vi "RandomPointEnemyField.vi"(9 "Field defense":dbl[](array[numeric]), 10 "IA State Input":T1) -> (2 "Point Enemy Field":dbl[](array[numeric]))   [LabVIEW 2017]
uses:
  Core/AI Input.ctl
  Core/AI Robot.ctl
  Intel/Functions Enum.ctl
  Intel/AttackerStates.ctl
  Path Planning/RRT/PathDests.ctl
  Path Planning/RRT/PathDest.ctl
  Core/AI Ball.ctl
  Core/Field Size.ctl
  Core/AI Judge.ctl
  Intel/Command Enum.ctl
  Util/Events/Events.ctl
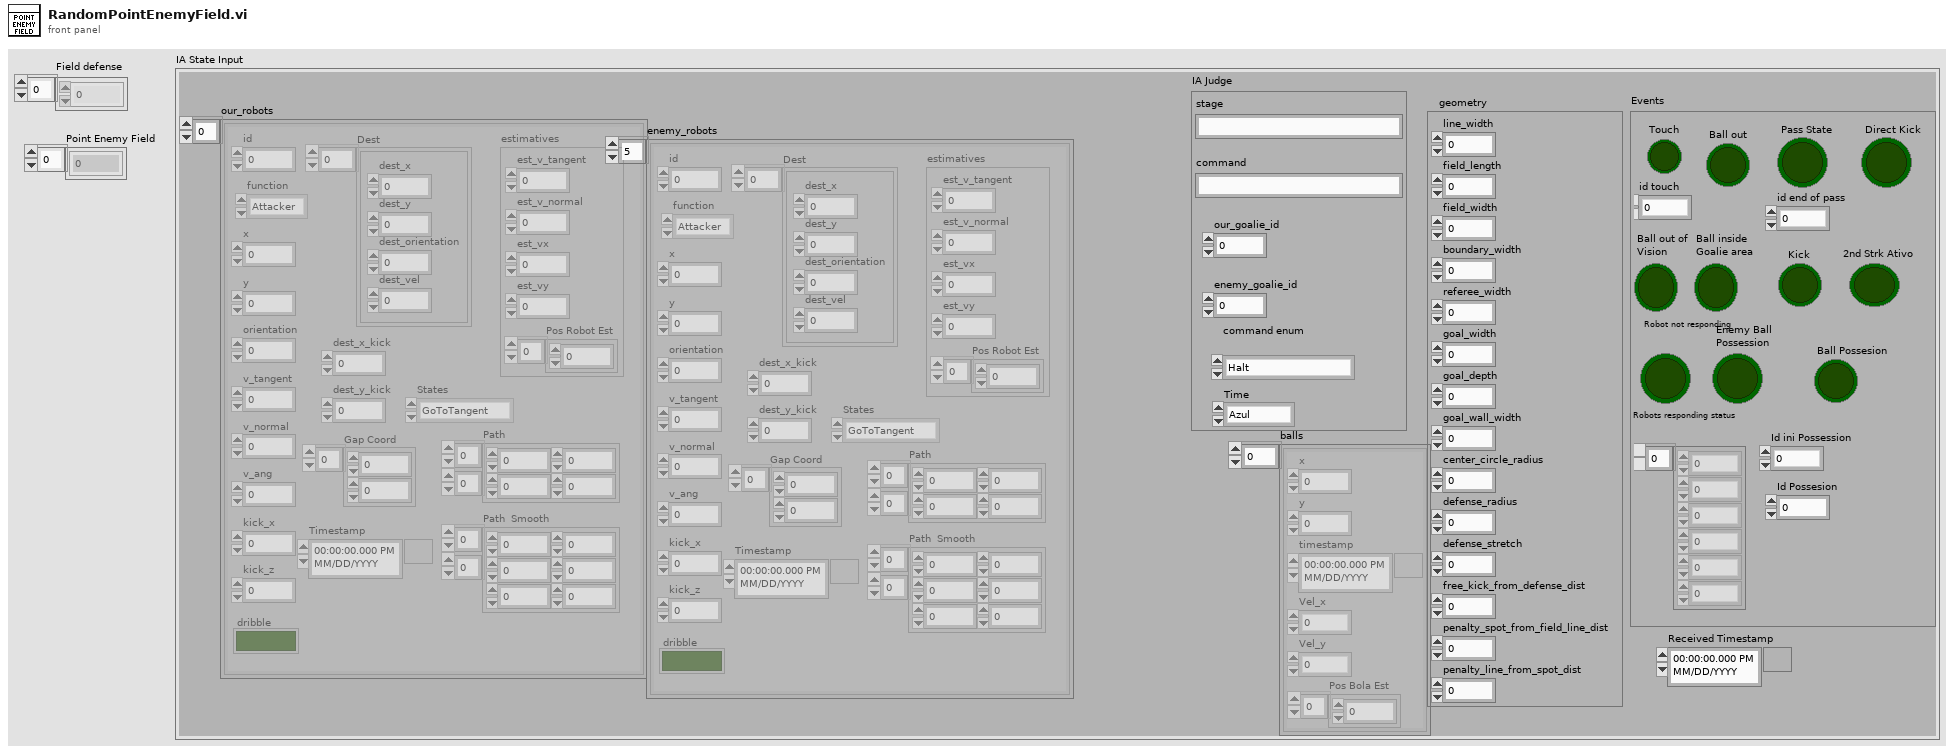
[diagram p1: front panel]
types:
  T1 = typedef "AI Input.ctl" = cluster{"our_robots":T2[], "enemy_robots":T2[], "balls":T7[], "geometry":T8, "IA Judge":T9, "Received Timestamp":timestamp, "Events":T11}
  T2 = typedef "AI Robot.ctl" = cluster{"id":u32, "function":T3, "x":dbl, "y":dbl, "orientation":dbl, "v_tangent":dbl, "v_normal":dbl, "v_ang":dbl, "kick_x":dbl, "kick_z":dbl, "dribble":bool, "Timestamp":timestamp, "estimatives":cluster{"est_v_tangent":dbl, "est_v_normal":dbl, "est_vx":dbl, "est_vy":dbl, "Pos Robot Est":dbl[]}, "dest_x_kick":dbl, "dest_y_kick":dbl, "Gap Coord":dbl[], "States":T4, "Path ":dbl[][], "Path  Smooth":dbl[][], "Dest":T5}
  T3 = typedef "Functions Enum.ctl" = enum16{"2nd Striker", "Attacker", "Goalie", "Defender", "Striker", "Goto 0", "Dummy", "Kicker", "ZigZag 0", "ZigZag 1", "ZigZag 2", "ZigZag 3", "ZigZag 4", "ZigZag 5", "ZigZag 6", "ZigZag 7", "ZigZag 8", ""}
  T4 = typedef "AttackerStates.ctl" = enum16{"Pass", "GoToTangent", "BallGetting", "GoToKick", ""}
  T5 = typedef "PathDests.ctl" = T6[]
  T6 = typedef "PathDest.ctl" = cluster{"dest_x":dbl, "dest_y":dbl, "dest_orientation":dbl, "dest_vel":dbl}
  T7 = typedef "AI Ball.ctl" = cluster{"x":dbl, "y":dbl, "timestamp":timestamp, "Vel_x":dbl, "Vel_y":dbl, "Pos Bola Est":dbl[]}
  T8 = typedef "Field Size.ctl" = cluster{"line_width":u32, "field_length":u32, "field_width":u32, "boundary_width":u32, "referee_width":u32, "goal_width":u32, "goal_depth":u32, "goal_wall_width":u32, "center_circle_radius":u32, "defense_radius":u32, "defense_stretch":u32, "free_kick_from_defense_dist":u32, "penalty_spot_from_field_line_dist":u32, "penalty_line_from_spot_dist":u32}
  T9 = typedef "AI Judge.ctl" = cluster{"stage":string, "command":string, "our_goalie_id":dbl, "enemy_goalie_id":dbl, "command enum":T10, "Time":enum16{"Azul", "Amarelo"}}
  T10 = typedef "Command Enum.ctl" = enum16{"Halt", "Stop", "Force Start", "PKA Normal Start", "Prepare Kickoff Ally", "PKE Normal Start", "Prepare Kickoff Enemy", "Prepare Penalty Ally", "PPA Normal Start", "Prepare Penalty Enemy", "PPE Normal Start", "Direct Free Enemy", "Direct Free Ally", "Indirect Free Enemy", "Indirect Free Ally", "Timeout Enemy", "Timeout Ally", "Goal Enemy", "Goal Ally", "Ball Placement Enemy", "Ball Placement Ally", "Normal Half Time", "Extra Time Break", "Extra Half Time", "None", "Post Game"}
  T11 = typedef "Events.ctl" = cluster{"Touch":bool, "Ball out":bool, "id touch":dbl, "Ball out of \nVision":bool, "Ball inside \nGoalie area":bool, "Robot not responding":bool, "Robots responding status":dbl[], "Enemy Ball \nPossession":bool, "Pass State":bool, "id end of pass":dbl, "Kick":bool, "Id ini Possession":dbl, "Ball Possesion":bool, "Id Possesion":dbl, "Direct Kick":bool, "2nd Strk Ativo":bool}
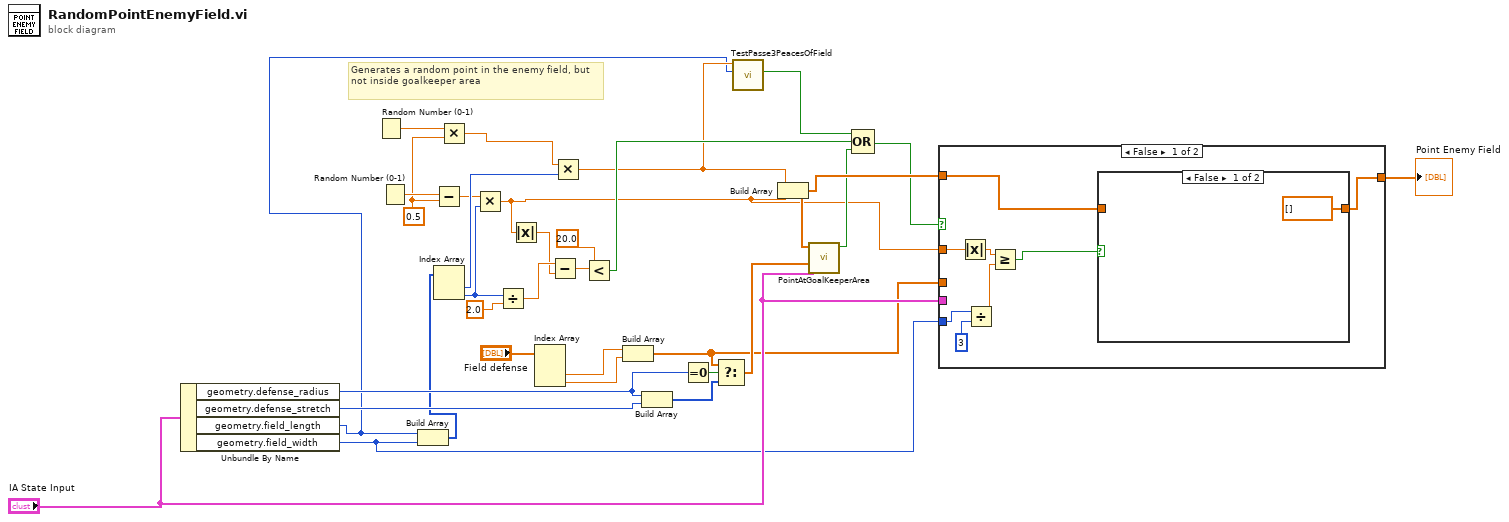
[diagram p0: block diagram]
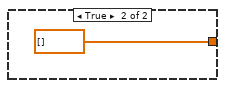
[diagram p3: hidden frame]
diagram:
  w29 = 0.5 ("y")
  # "Generates a random point in the enemy field, but not inside goalkeeper area"
  n1 = Unbundle By Name("IA State Input") -> ("geometry.defense_radius"=w14:u32, "geometry.defense_stretch"=w16:u32, "geometry.field_length"=w4:u32, "geometry.field_width"=w1:u32)
  n2 = Random Number (0-1)() -> (number: 0 to 1=w30:dbl)
  n3 = Random Number (0-1)() -> (number: 0 to 1=w31:dbl)
  n4 = Build Array(w4, w1) -> (w11:u32[])
  n5 = Subtract(x=w31, y=w29) -> (x-y=w32:dbl)
  n6 = Index Array(array=w11) -> (element #1=w33:u32, element #2=w26:u32)  [unwired: 2 in]
  n7 = Multiply(x=w30, y=w29) -> (x*y=w6:dbl)
  n8 = Multiply(x=w32, y=w26) -> (x*y=w2:dbl)
  n9 = Divide(x=w26, y=2.0) -> (x/y=w24:dbl)
  n10 = Absolute Value(x=w2) -> (abs(x)=w23:dbl)
  n11 = Index Array(array="Field defense") -> (element #2=w9:dbl, element #3=w8:dbl)  [unwired: 3 in, 1 out]
  n12 = Subtract(x=w24, y=w23) -> (x-y=w22:dbl)
  n13 = Multiply(x=w6, y=w33) -> (x*y=w5:dbl)
  n14 = Less?(x=w22, y=20.0) -> (x < y?=w19:bool)
  n15 = Build Array(w9, w8) -> (w7:dbl[])
  n16 = Build Array(w14, w16) -> (w13:u32[])
  n17 = Equal To 0?(x=w14) -> (x = 0?=w15:bool)
  n18 = Select(t=w7, s=w15, f=w13) -> (s? t:f=w12:dbl[])
  n19 = call "TestPasse3PeacesOfField.vi"("Field Length"=w4, "X"=w5) -> ("Segundo Terço"=w3:bool)  [unwired: 7 in, 2 out]
  n20 = Build Array(w5, w2) -> (w28:dbl[])
  n21 = call "PointAtGoalKeeperArea.vi"("Field defense"=w12, "IA State Input"="IA State Input", "Array"=w28) -> ("Point inside goalkeeper area ?"=w20:bool)  [unwired: 8 in]
  n22 = Compound Arithmetic op=OR(w3, w19, w20) -> (w18:bool)
  n23 = case shown="False" w18 {
    tunnel: [w41 dbl[] []] -> w27
    tunnel: w28 -> [w40 _]
    tunnel: "IA State Input" -> [_ _]
    tunnel: w7 -> [_ _]
    tunnel: w2 -> [w39 _]
    tunnel: w1 -> [w36 _]
    frame False {
      n24 = Absolute Value(x=w39) -> (abs(x)=w38:dbl)
      n25 = Divide(x=w36, y=u32 3) -> (x/y=w37:dbl)
      n26 = Greater Or Equal?(x=w38, y=w37) -> (x >= y?=w34:bool)
      n27 = case shown="False" w34 {
        tunnel: [dbl[] [] w43] -> w41
        tunnel: w40 -> [_ w43]
        frame False {
        }
        frame True {
        }
      }
    }
    frame True {
    }
  }
  "Point Enemy Field" <- w27
